vi "Set Log Specification Type.vi"(8 "error in (no error)":errorcluster, 10 "Log Specification Type":T1, 11 "Log File Specification in":refnum<class "Log File Specification.lvclass">) -> (0 "error out":errorcluster, 3 "Log File Specification out":refnum<class "Log File Specification.lvclass">)   [LabVIEW 2012, in "Waveform Data Logger Shared.lvlib" / "Log File Specification.lvclass"]
uses:
  Log File Specification.lvclass
  Log Specification Type.ctl
  Log File Specification.lvclass/Log File Specification.ctl
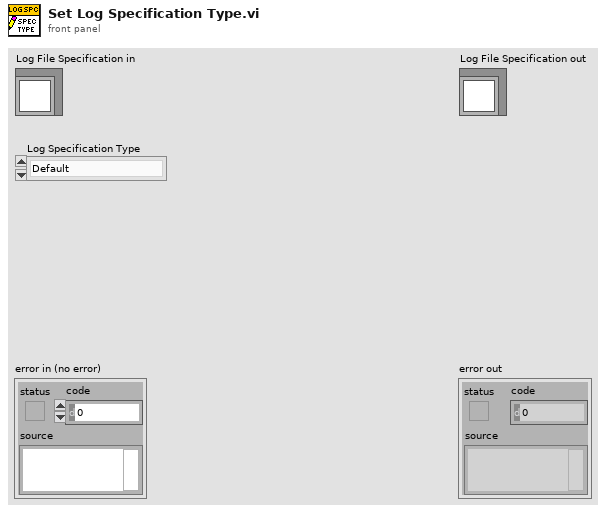
[diagram p1: front panel]
types:
  T1 = typedef "Waveform Data Logger Shared.lvlib/Log File Specification.lvclass/Log Specification Type.ctl" = enum16{"Default", "TDMS", "Text", "Waveform TDMS"}
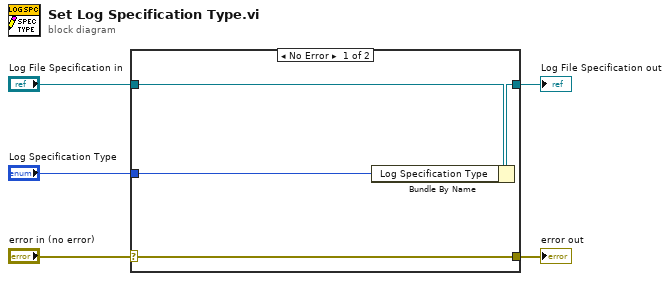
[diagram p0: block diagram]
diagram:
  n1 = case shown="No Error" "error in (no error)" {
    selector: "error in (no error)" -> [w9 w10]
    tunnel: [w9 w10] -> w4
    tunnel: [w7 w11] -> w2
    tunnel: "Log File Specification in" -> [w8 w11]
    tunnel: "Log Specification Type" -> [w6 _]
    frame No Error {
      n2 = Bundle By Name(cluster=w8, "Log Specification Type"=w6) -> (w7:refnum<class "Log File Specification.lvclass">)
    }
    frame Error {
    }
  }
  "error out" <- w4
  "Log File Specification out" <- w2
